vi "eFGV - Logout.vi"(6 "Action":T1, 8 "Error In":errorcluster, 11 "Logout In":bool) -> (0 "Error Out":errorcluster, 2 "Event Logout":refnum<user-event>, 3 "Logout Out":bool)   [LabVIEW 2020]
uses:
  Control/State - eFGV.ctl
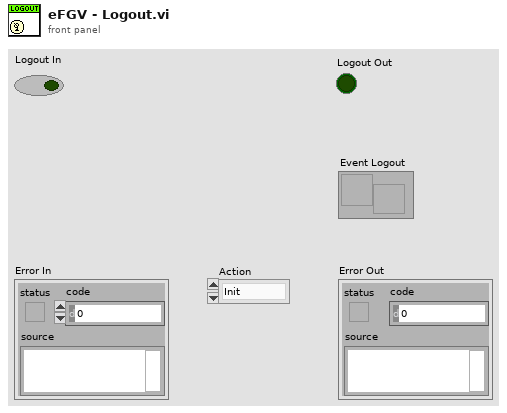
[diagram p1: front panel]
types:
  T1 = typedef "State - eFGV.ctl" = enum16{"Init", "Read", "Write", "Exit"}
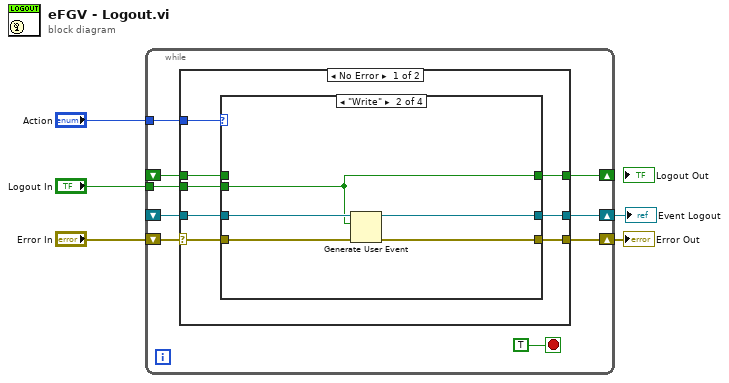
[diagram p0: block diagram]
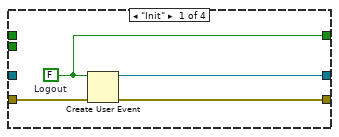
[diagram p2: hidden frame]
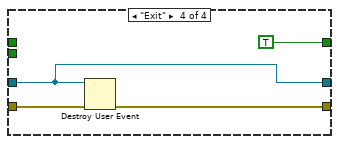
[diagram p4: hidden frame]
diagram:
  n1 = while {
    tunnel: "Action" -> [w11]
    shift-right: [w14] -> w5
    shift-left: "Error In" -> [w13]
    shift-right: [w10] -> w1
    shift-left: _ -> [w9]
    tunnel: "Logout In" -> [w8]
    shift-right: [w7] -> _
    shift-left: _ -> [w6]
    stop <- TRUE stop-if-true
    n2 = case shown="No Error" w13 {
      selector: w13 -> [w21 w41]
      tunnel: [w22 w41] -> w14
      tunnel: w11 -> [w20 _]
      tunnel: [w19 w39] -> w10
      tunnel: w9 -> [w18 w39]
      tunnel: w8 -> [w17 _]
      tunnel: [w16 w40] -> w7
      tunnel: w6 -> [w15 w40]
      frame No Error {
        n3 = case shown="\"Write\"" w20 {
          tunnel: w21 -> [w26 w31 w34 w38]
          tunnel: [w25 w30 w34 w37] -> w22
          tunnel: [w24 w27 w33 w35] -> w19
          tunnel: w18 -> [_ w29 w33 w35]
          tunnel: w17 -> [_ w28 _ _]
          tunnel: [w23 w28 w32 TRUE ("Stop?")] -> w16
          tunnel: w15 -> [_ _ w32 _]
          frame "Init" {
            w23 = FALSE  # Logout
            n4 = Create User Event(user event datatype=w23, error in=w26) -> (user event=w24:refnum<user-event>, error out=w25:errorcluster)
          }
          frame "Write" {
            n5 = Generate User Event(user event=w29, event data cluster=w28, error in=w31) -> (user event out=w27:refnum<user-event>, error out=w30:errorcluster)  [unwired: 1 in]
          }
          frame "Read" {
          }
          frame "Exit" {
            n6 = Destroy User Event(user event=w35, error in=w38) -> (error out=w37:errorcluster)
          }
        }
      }
      frame Error {
      }
    }
  }
  "Error Out" <- w5
  "Event Logout" <- w1
